vi "GLIMPSE Splash Screen.vi"() -> ()   [LabVIEW 2016]
uses:
  GLIMPSE Globals.vi
panel:
  out "String":string="GLIMPSE v. 35 (2/04)"
  # "https://github.com/gelles-brandeis/Glimpsel\n\nCopyright (c) 1999-20010,2011,2012,,2013,2014\n by Jeff Gelles, Brandeis Univ.\nThis is licensed software: \nClick on the \"About Glimpse\" button for details."
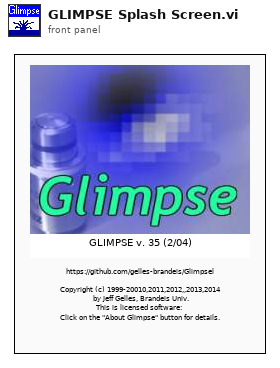
[diagram p1: front panel]
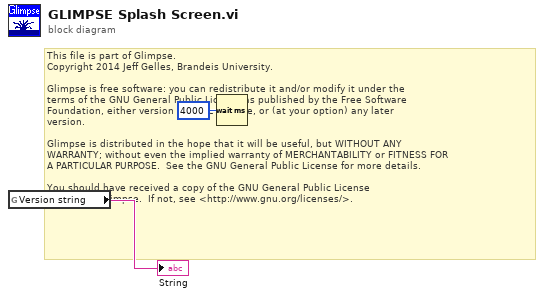
[diagram p0: block diagram]
diagram:
  # "This file is part of Glimpse. \nCopyright 2014 Jeff Gelles, Brandeis University.    \n\nGlimpse is free software: you can redistribute it and/or modify it under the \nterms of the GNU General Public License as published by the Free Software \nFoundation, either version 3 of the License, or (at your option) any later \nversion.\n\nGlimpse is distributed in the hope that it will be useful, but WITHOUT ANY \nWARRANTY; without even the implied warranty of MERCHANTABILITY or FITNESS FOR \nA PARTICULAR PURPOSE.  See the GNU General Public License for more details.\n\nYou should have received a copy of the GNU General Public License\nalong with Glimpse.  If not, see <http://www.gnu.org/licenses/>."
  n1 = global read "GLIMPSE Globals.vi" "Version string"() -> (→"String":string)
  n2 = Wait (ms)(milliseconds to wait=u32 4000) -> ()  [unwired: 1 out]
